vi "Go to Work State.vi"(8 "error in (no error)":errorcluster, 11 "Chef UI in":refnum<class "Chef UI.lvclass">) -> (0 "error out":errorcluster, 3 "Chef UI out":refnum<class "Chef UI.lvclass">)   [LabVIEW 2024, in "Chef UI.lvlib" / "Chef UI.lvclass"]
uses:
  Chef UI.lvclass
  Chef UI.lvclass/Chef UI.ctl
  Chef State/Chef State Messages/Go to Work Msg/Go to Work Msg.lvclass
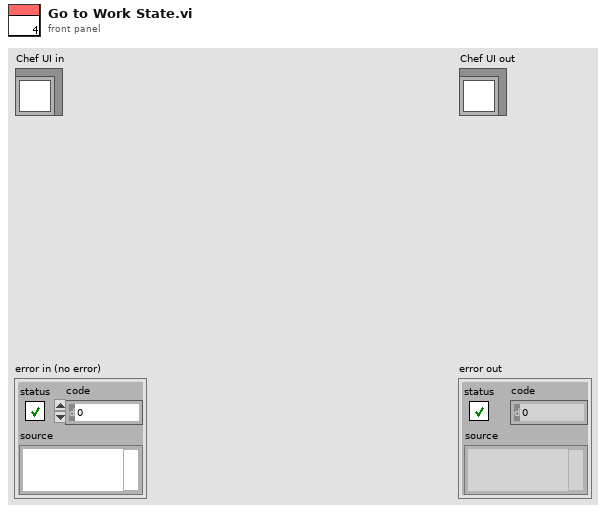
[diagram p1: front panel]
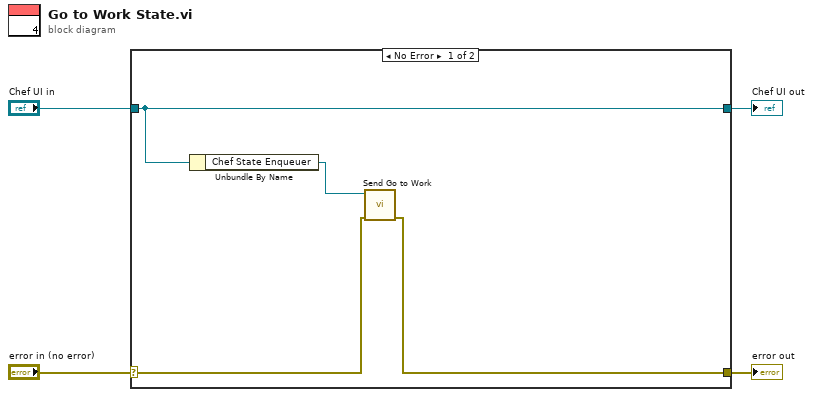
[diagram p0: block diagram]
diagram:
  n1 = case shown="No Error" "error in (no error)" {
    selector: "error in (no error)" -> [w6 w10]
    tunnel: [w5 w10] -> w3
    tunnel: [w8 w9] -> w1
    tunnel: "Chef UI in" -> [w8 w9]
    frame No Error {
      n2 = Unbundle By Name(w8) -> ("Chef State Enqueuer"=w7:refnum<class "Message Enqueuer.lvclass">)
      n3 = call "Send Go to Work.vi"("error in (no error)"=w6, "Message Enqueuer"=w7) -> ("error out"=w5:errorcluster)  [unwired: 8 in, 1 out]
    }
    frame Error {
    }
  }
  "error out" <- w3
  "Chef UI out" <- w1
